vi "dV-dI and Crit-Current.vi"(5 "V offset":dbl, 6 "I offset":dbl, 7 "How many V sweep periods?":dbl=1.0, 8 "Input data":cluster{dbl[], dbl[]}(graph), 9 "dV/dI (Ic) Parameters":T2={"High current value"=7e-09, "Low currentvalue"=-7e-09, "decimation points"=600, "side points"=8, "polynomial order 2"=3, "peak width"=18, "peak threshold"=75000.0, "trough threshold"=55000.0}) -> (0 "Ave Critical Current":dbl=1.3533333333333336e-09, 1 "Ic's":T1={"Ic (+) (A)"=1.400000000000001e-09, "Ic (-) (A)"=-1.3066666666666663e-09, "Ic (average) (A)"=1.3533333333333336e-09} {"Ic (+) (A)" format="%#_6p"; "Ic (-) (A)" format="%#_6p"; "Ic (average) (A)" format="%#_6p"}, 2 "dV/dI and Ic peaks":cluster{"X Subset":dbl[], "Filtered X":dbl[]}[](graph), 3 "V vs I - Offset Plot":cluster{dbl[], dbl[]}[](graph), 4 "Data for second derivative":cluster{"xi used":dbl[], "dX/dt":dbl[]})   [LabVIEW 2016]
uses:
  <vilib>/Analysis/3filter.llb/Savitzky-Golay Filter (DBL).vi
  <vilib>/Analysis/NI_AALPro.lvlib
  <vilib>/gmath/NI_Gmath.lvlib
  <vilib>/Analysis/NI_AALBase.lvlib
  <vilib>/Analysis/NI_AAL_SigProc.lvlib
panel:
  out "High current value":dbl=7e-09
  out "Low currentvalue":dbl=-7e-09
  out "decimation points":i32=600
  out "side points":i32=8
  out "polynomial order 2":i32=3
  out "peak width":i32=18
  out "peak threshold":dbl=75000.0
  out "trough threshold":dbl=55000.0
  # "paste data here"
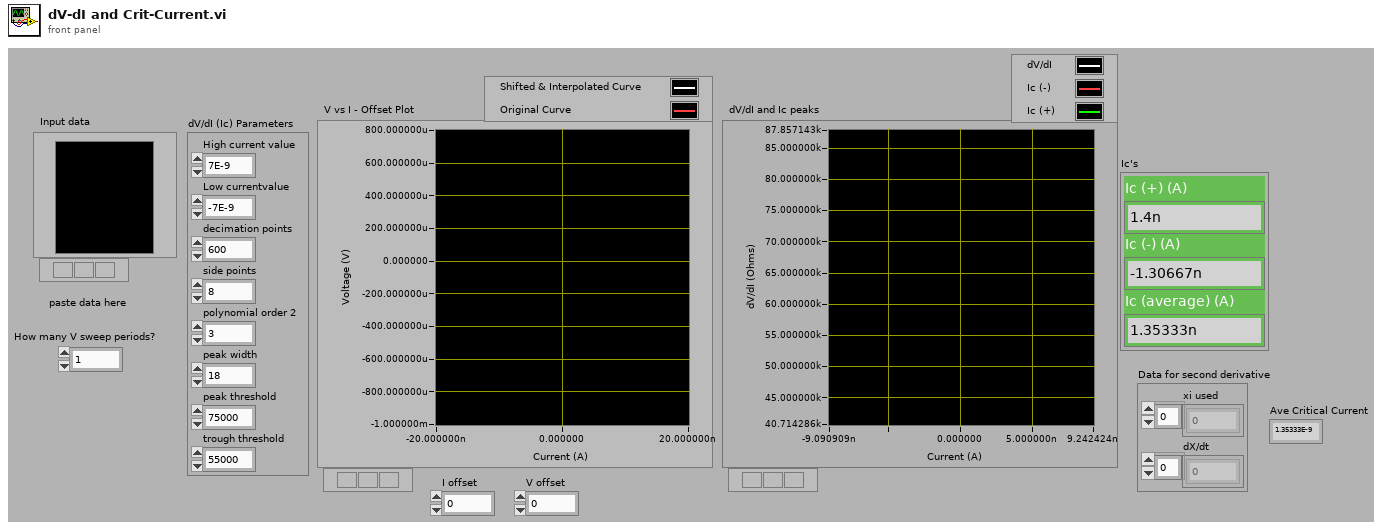
[diagram p1: front panel]
types:
  T1 = cluster{"Ic (+) (A)":dbl, "Ic (-) (A)":dbl, "Ic (average) (A)":dbl}
  T2 = cluster{"High current value":dbl, "Low currentvalue":dbl, "decimation points":i32, "side points":i32, "polynomial order 2":i32, "peak width":i32, "peak threshold":dbl, "trough threshold":dbl}
  T3 = cluster{"Positive Val":dbl, "Negative Val":dbl, "Ave Ic":dbl}
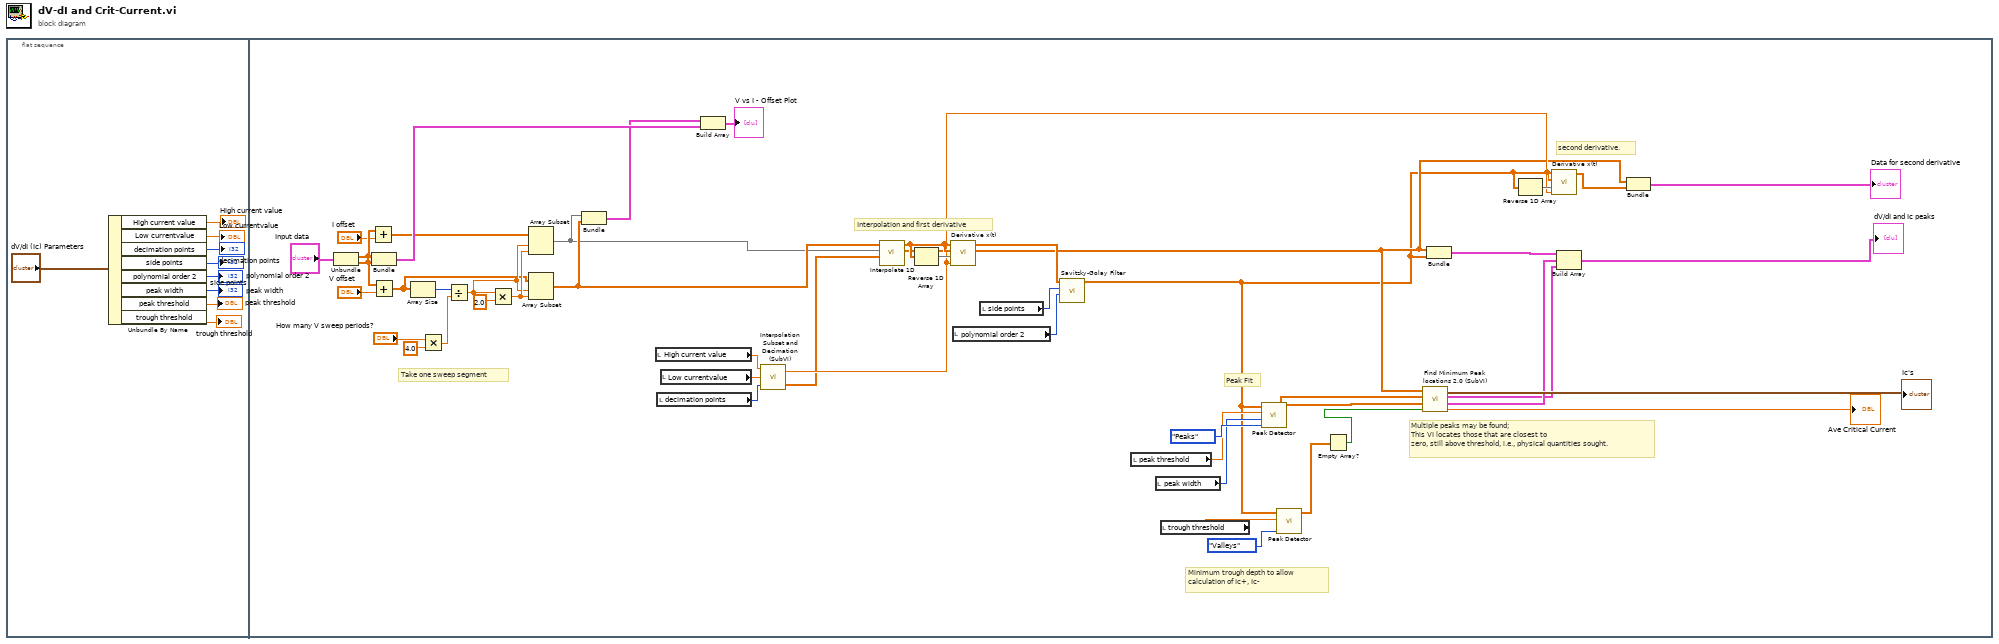
[diagram p0: block diagram]
diagram:
  n1 = flat-sequence {
    frame #0 {
      n2 = Unbundle By Name("dV/dI (Ic) Parameters") -> ("High current value"=→"High current value":dbl, "Low currentvalue"=→"Low currentvalue":dbl, "decimation points"=→"decimation points":i32, "side points"=→"side points":i32, "polynomial order 2"=→"polynomial order 2":i32, "peak width"=→"peak width":i32, "peak threshold"=→"peak threshold":dbl, "trough threshold"=→"trough threshold":dbl)
    }
    frame #1 {
      # "second derivative."
      # "Multiple peaks may be found;\nThis VI locates those that are closest to\nzero, still above threshold, i.e., physical quantities sought."
      # "Minimum trough depth to allow \ncalculation of Ic+, Ic-"
      # "Peak Fit"
      # "Interpolation and first derivative"
      # "Take one sweep segment"
      n3 = Unbundle("Input data") -> (w56:dbl[], w57:dbl[])
      n4 = Add(x=w56, y="I offset") -> (x+y=w43:dbl[])
      n5 = Bundle(w56, w57) -> (w58:cluster{dbl[], dbl[]})  [unwired: 1 in]
      n6 = Add(x=w57, y="V offset") -> (x+y=w50:dbl[])
      n7 = Array Size(array=w50) -> (size(s)=w46:i32)
      n8 = Multiply(x="How many V sweep periods?", y=4.0) -> (x*y=w47:dbl)
      n9 = Divide(x=w46, y=w47) -> (x/y=w51:dbl)
      n10 = Multiply(x=w51, y=2.0) -> (x*y=w52:dbl)
      n11 = Array Subset(array=w43, index=w51, length=w52) -> (w53:dbl[])
      n12 = Array Subset(array=w50, index=w51, length=w52) -> (w54:dbl[])
      n13 = Bundle(w53, w54) -> (w55:cluster{dbl[], dbl[]})  [unwired: 1 in]
      n14 = local read "High current value"() -> (w14:dbl)
      n15 = local read "decimation points"() -> (w12:i32)
      n16 = local read "Low currentvalue"() -> (w13:dbl)
      n17 = Build Array(w55, w58) -> (→"V vs I - Offset Plot":cluster{dbl[], dbl[]}[])
      n18 = call "Interpolation Subset and Decimation (SubVI).vi"("decimation points"=w12, "Low value"=w13, "High value"=w14) -> ("Points to use in interpolation (xi)"=w25:dbl[], "Numeric"=w26:dbl)
      n19 = call <vilib>:"Interpolate 1D.vi"("xi"=w25, "X"=w53, "Y"=w54) -> ("xi used"=w20:dbl[], "yi"=w37:dbl[])  [unwired: 6 in, 1 out]
      n20 = Reverse 1D Array(array=w37) -> (reversed array=w38:dbl[])
      n21 = call <vilib>:"Derivative x(t).vi"("dt"=w26, "Final Condition"=w38, "Initial Condition"=w37, "X"=w37) -> ("dX/dt"=w36:dbl[])  [unwired: 6 in, 1 out]
      n22 = local read "polynomial order 2"() -> (w16:i32)
      n23 = local read "side points"() -> (w15:i32)
      n24 = call-poly <vilib>:"Savitzky-Golay Filter.vi"("polynomial order"=w16, "side points"=w15, "X"=w36) -> ("Filtered X"=w10:dbl[])  [unwired: 7 in, 1 out]
      n25 = local read "peak threshold"() -> (w18:dbl)
      n26 = local read "peak width"() -> (w17:i32)
      n27 = local read "trough threshold"() -> (w19:dbl)
      n28 = call <vilib>:"Peak Detector.vi"("peaks/valleys"=enum32{"Peaks", "Valleys"}."Peaks", "width"=w17, "threshold"=w18, "X"=w10) -> ("Amplitudes"=w28:dbl[], "Locations"=w27:dbl[])  [unwired: 3 in, 3 out]
      n29 = call <vilib>:"Peak Detector.vi"("peaks/valleys"=enum32{"Peaks", "Valleys"}."Valleys", "threshold"=w19, "X"=w10) -> ("Locations"=w34:dbl[])  [unwired: 4 in, 4 out]
      n30 = Empty Array?(array=w34) -> (empty?=w35:bool)
      n31 = call "Find Minimum Peak locations 2.0 (SubVI).vi"("Empty Array?"=w35, "Amplitudes"=w28, "Locations"=w27, "X Array"=w20) -> ("Ave Critical Current"=→"Ave Critical Current":dbl, "Negative Location"=w30:cluster{dbl[], dbl[]}, "Positive Location"=w29:cluster{dbl[], dbl[]}, "Ic's"=→"Ic's":T3)
      n32 = Bundle("xi used"=w20, "Filtered X"=w10) -> (w24:cluster{"xi used":dbl[], "Filtered X":dbl[]})  [unwired: 1 in]
      n33 = Reverse 1D Array(array=w10) -> (reversed array=w39:dbl[])
      n34 = call <vilib>:"Derivative x(t).vi"("dt"=w26, "Final Condition"=w39, "Initial Condition"=w10, "X"=w10) -> ("dX/dt"=w40:dbl[])  [unwired: 6 in, 1 out]
      n35 = Build Array(w24, w30, w29) -> (→"dV/dI and Ic peaks":cluster{"xi used":dbl[], "Filtered X":dbl[]}[])
      n36 = Bundle("xi used"=w20, "dX/dt"=w40) -> (→"Data for second derivative":cluster{"xi used":dbl[], "dX/dt":dbl[]})  [unwired: 1 in]
    }
  }
